vi "Active Noise Control (FPGA).vi"() -> ()   [LabVIEW 2023]
doc: "This VI runs on an FPGA target. This VI uses a fixed-point LMS adaptive filter to identify the impulse response of the secondary path, acquires noise at the location of interest with the error microphone, and uses a filtered-X LMS adaptive filter to generate a control waveform for the control speaker. This VI assumes you know the frequency of the monotone primary noise and uses this frequency to generate the primary noise as the input of the adaptive filter."
uses:
  <vilib>/eio/EIONode/EIONode.xnode
  <vilib>/rvi/FXPMathLib/FxpAdd/XNode/nifxpmath_Add.xnode
  <vilib>/rvi/FXPMathLib/FxpSinAndCos/XNode/nifxpmath_SinAndCos.xnode
  <vilib>/rvi/FXPMathLib/FxpDiv/XNode/nifxpmath_Div.xnode
  <vilib>/eio/EIOPropertyNode/EIOPropertyNode.xnode
  <vilib>/LabVIEW Targets/FPGA/cRIO/shared/nicrio_ModuleControls/nicrio_cRIO-9233_DataRatesRing.ctl
  <vilib>/rvi/DataTransferAndStorage/Container/XNode/niFpgaContainer.xnode
  <vilib>/rvi/FXPMathLib/FxpDiv/simVIs/DllFxpDivTemp_sub.vi
  <vilib>/rvi/FXPMathLib/FxpDiv/subVIs/nifxpmath_Div_SimConfig.ctl
  <vilib>/rvi/FXPMathLib/FxpSinAndCos/simVIs/DllFxpSinAndCosTemp_sub.vi
  <vilib>/rvi/FXPMathLib/FxpSinAndCos/subVIs/nifxpmath_SinAndCos_SimConfig.ctl
  <vilib>/rvi/eio/common/nirviEmuTemplateMethod_errors.vi
  <vilib>/rvi/eio/common/nirviEmuTemplatePropertyGet_errors.vi
  <vilib>/rvi/eio/common/nirviEmuTemplatePropertyGet_noerrors.vi
  <vilib>/rvi/eio/common/nirviEmuTemplatePropertySet_errors.vi
  <vilib>/rvi/eio/common/nirviEmuTemplatePropertySet_noerrors.vi
  <vilib>/rvi/interface/RandomDataEmulation/nirviRandomDataFpgaReadWriteTemplate.vi
  <vilib>/rvi/Memory/Memory_Emulation/nirvimemoryEmulation.vi
  <vilib>/rvi/Memory/Memory_Emulation/nirvimemoryFastEmulation.vi
  <vilib>/rvi/FXPMathLib/sim/FxpSim.dll
panel:
  in  "frequency (Hz)":fxp<+/-,16,16>
  in  "reset":bool
  in  "control on":bool
  in  "stop":bool
  in  "step size (FXLMS)":fxp<+/-,16,-2>
  in  "gain for microphone channel":i32
  in  "step size (LMS)":fxp<+/-,16,-5>
  in  "stop modeling":bool
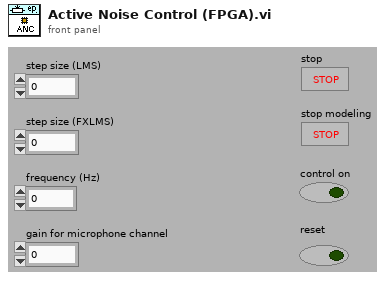
[diagram p1: front panel]
types:
  T1 = typedef "nicrio_cRIO-9233_DataRatesRing.ctl" = u8
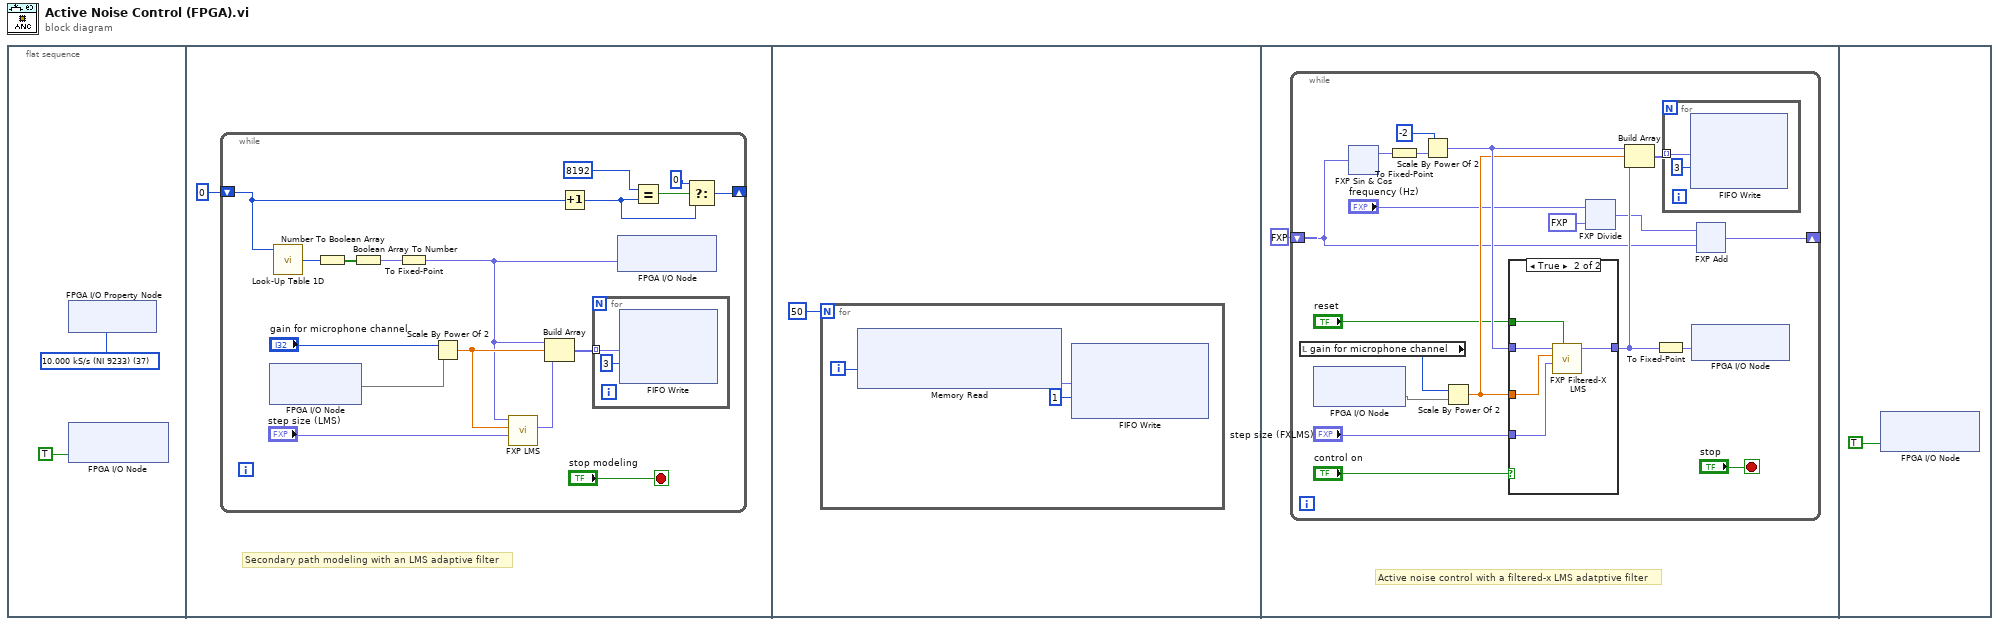
[diagram p0: block diagram]
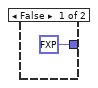
[diagram p2: hidden frame]
diagram:
  n1 = flat-sequence {
    frame #0 {
      w1 = T1 37 items=["50.000 kS/s (NI 9233)"=2, "33.333 kS/s (NI 9233)"=3, "25.000 kS/s (NI 9233)"=34, "16.667 kS/s (NI 9233)"=35, "12.500 kS/s (NI 9233)"=36, "10.000 kS/s (NI 9233)"=37, "  8.333 kS/s (NI 9233)"=38, "  7.143 kS/s (NI 9233)"=39, "  6.250 kS/s (NI 9233)"=40, "  5.556 kS/s (NI 9233)"=41, "  5.000 kS/s (NI 9233)"=42, "  4.545 kS/s (NI 9233)"=43, "  4.167 kS/s (NI 9233)"=44, "  3.846 kS/s (NI 9233)"=45, "  3.571 kS/s (NI 9233)"=46, "  3.333 kS/s (NI 9233)"=47, "  3.125 kS/s (NI 9233)"=48, "  2.941 kS/s (NI 9233)"=49, "  2.778 kS/s (NI 9233)"=50, "  2.632 kS/s (NI 9233)"=51, "  2.500 kS/s (NI 9233)"=52, "  2.381 kS/s (NI 9233)"=53, "  2.273 kS/s (NI 9233)"=54, "  2.174 kS/s (NI 9233)"=55, "  2.083 kS/s (NI 9233)"=56, "  2.000 kS/s (NI 9233)"=57] ("Data Rate")
      n2 = xnode "FPGA I/O Property Node"("Data Rate"=w1) -> ()  [unwired: 1 in, 1 out]
      n3 = xnode "FPGA I/O Node"("Mod1/Start"=TRUE) -> ()  [unwired: 2 in, 2 out]
    }
    frame #1 {
      # "Secondary path modeling with an LMS adaptive filter"
      n4 = while {
        shift-right: [w15] -> _
        shift-left: u16 0 -> [w17]
        stop <- "stop modeling" stop-if-true
        n5 = xnode "FPGA I/O Node"() -> ("Mod1/AI0"=w12)  [unwired: 2 in, 2 out]
        n6 = call "Look-Up Table 1D"("address"=w17) -> ("data out"=w14:i16)  [unwired: 8 in]
        n7 = Number To Boolean Array(number=w14) -> (Boolean array=w13:bool[])
        n8 = Boolean Array To Number(Boolean array=w13) -> (number=w10:fxp<+/-,16,1>)
        n9 = To Fixed-Point(number=w10) -> (fixed-point=w4:fxp<+/-,24,4>)  [unwired: 1 out]
        n10 = Scale By Power Of 2(n="gain for microphone channel", x=w12) -> (x*2^n=w9:dbl)
        n11 = call "FXP LMS.vi"("step size"="step size (LMS)", "d(n)"=w9, "x(n)"=w4) -> ("e(n)"=w8:fxp<+/-,24,4>)  [unwired: 1 in, 7 out]
        n12 = Build Array(w4, w9, w8) -> (w7:fxp<+/-,24,4>[])
        n13 = Increment(x=w17) -> (x+1=w5:u16)
        n14 = for {
          tunnel: w7 -> [w21] mode=indexing
          n15 = xnode ("FIFO Write")("Element"=w21, "Timeout"=3) -> ()  [unwired: 1 in, 2 out]
        }
        n16 = xnode "FPGA I/O Node"("Mod2/AO0"=w4) -> ()  [unwired: 1 in, 1 out]
        n17 = Equal?(x=u16 8192 ("y"), y=w5) -> (x = y?=w18:bool)
        n18 = Select(t=u16 0, s=w18, f=w5) -> (s? t:f=w15:u16)
      }
    }
    frame #2 {
      n19 = for {
        N: 50 -> [_]
        i -> [w25]
        n20 = xnode ("Memory Read")("Address"=w25) -> ("Data"=w24:fxp<+/-,24,4>)  [unwired: 1 in, 1 out]
        n21 = xnode ("FIFO Write")("Element"=w24, "Timeout"=1) -> ()  [unwired: 1 in, 2 out]
      }
    }
    frame #3 {
      # "Active noise control with a filtered-x LMS adatptive filter"
      n22 = while {
        shift-right: [w33] -> _
        shift-left: fxp<+/-,32,1> -1.0 -> [w30]
        stop <- "stop" stop-if-true
        n23 = local read "gain for microphone channel"() -> (w45:i32)
        n24 = xnode "FPGA I/O Node"() -> ("Mod1/AI0"=w46)  [unwired: 2 in, 2 out]
        n25 = xnode "FXP Sin & Cos"("x (pi)"=w30) -> ("sin(x)"=w31:fxp<+/-,16,2>)  [unwired: 1 out]
        n26 = To Fixed-Point(number=w31) -> (fixed-point=w32:fxp<+/-,24,4>)  [unwired: 1 out]
        n27 = Scale By Power Of 2(n=-2, x=w32) -> (x*2^n=w42:fxp<+/-,24,4>)
        n28 = Scale By Power Of 2(n=w45, x=w46) -> (x*2^n=w37:dbl)
        n29 = case shown="True" "control on" {
          tunnel: "step size (FXLMS)" -> [_ w109]
          tunnel: w42 -> [_ w108]
          tunnel: w37 -> [_ w107]
          tunnel: [fxp<+/-,24,4> 0.0 w105] -> w40
          tunnel: "reset" -> [_ w106]
          frame False {
          }
          frame True {
            n30 = call "FXP Filtered-X LMS.vi"("reset"=w106, "step size"=w109, "e(n)"=w107, "x(n)"=w108) -> ("y(n)"=w105:fxp<+/-,24,4>)  [unwired: 1 in, 6 out]
          }
        }
        n31 = xnode "FXP Divide"("x"="frequency (Hz)", "y"=fxp<+/-,16,16> 5000.0) -> ("x/y"=w29:fxp<+/-,32,1>)
        n32 = Build Array(w42, w37, w40) -> (w43:fxp<+/-,24,4>[])
        n33 = To Fixed-Point(number=w40) -> (fixed-point=w41:fxp<+/-,20,5>)  [unwired: 1 out]
        n34 = for {
          tunnel: w43 -> [w110] mode=indexing
          n35 = xnode ("FIFO Write")("Element"=w110, "Timeout"=3) -> ()  [unwired: 1 in, 2 out]
        }
        n36 = xnode "FPGA I/O Node"("Mod2/AO0"=w41) -> ()  [unwired: 1 in, 1 out]
        n37 = xnode "FXP Add"("x"=w29, "y"=w30) -> ("x+y"=w33:fxp<+/-,32,1>)
      }
    }
    frame #4 {
      n38 = xnode "FPGA I/O Node"("Mod1/Stop"=TRUE) -> ()  [unwired: 2 in, 2 out]
    }
  }
